vi "Analysis.TestSizeVariant.vi"() -> ()   [LabVIEW 2024]
panel:
  out "Variant":variant
  out "Dur(s)":dbl
  out "Cnt":i32
  out "i":i32
  in  "Count":i32=100000
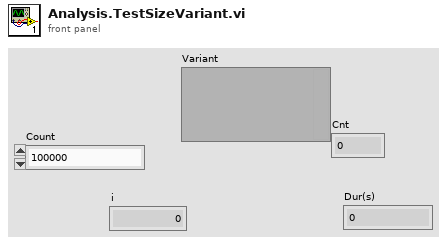
[diagram p1: front panel]
types:
  T1 = cluster{"Bool":bool, "Int":i32, "Num":dbl, "Str":string, "Name":string}
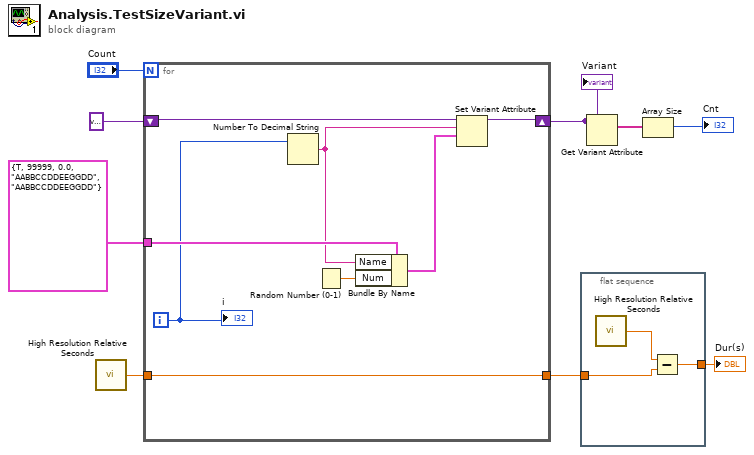
[diagram p0: block diagram]
diagram:
  n1 = call <vilib>:"High Resolution Relative Seconds.vi"() -> ("relative seconds"=w3:dbl)
  n2 = for {
    N: "Count" -> [_]
    shift-right: [w16] -> w7
    shift-left: variant -> [w17]
    tunnel: T1 {"Bool"=TRUE, "Int"=99999, "Num"=0.0, "Str"="AABBCCDDEEGGDD", "Name"="AABBCCDDEEGGDD"} -> [w14]
    tunnel: w3 -> [w12]
    tunnel: [w12] -> w2
    i -> [w11]
    n3 = Number To Decimal String(number=w11) -> (decimal integer string=w13:string)  [unwired: 1 in]
    n4 = Random Number (0-1)() -> (number: 0 to 1=w15:dbl)
    n5 = Bundle By Name(cluster=w14, "Name"=w13, "Num"=w15) -> (w10:T1)
    n6 = Set Variant Attribute(Variant=w17, name=w13, value=w10) -> (Variant out=w16:variant)  [unwired: 1 in, 2 out]
    "i" <- w11
  }
  "Variant" <- w7
  n7 = flat-sequence {
    tunnel: w2 -> [w19]
    tunnel: [w18] -> w1
    frame #0 {
      n8 = call <vilib>:"High Resolution Relative Seconds.vi"() -> ("relative seconds"=w20:dbl)
      n9 = Subtract(x=w20, y=w19) -> (x-y=w18:dbl)
    }
  }
  n10 = Get Variant Attribute(Variant=w7) -> (names=w6:string[])  [unwired: 3 in, 3 out]
  n11 = Array Size(array=w6) -> (size(s)=→"Cnt":i32)
  "Dur(s)" <- w1
